vi "相对偏差百分比出数.vi"(0 "基准值":dbl, 2 "原始值":dbl, 3 "相对偏差百分比":dbl) -> (6 "取值输出":dbl, 7 "随机数？":bool)   [LabVIEW 2016, in "random number.lvlib"]
uses:
  random number.lvlib
panel:
  out "下限":dbl
  out "上限":dbl
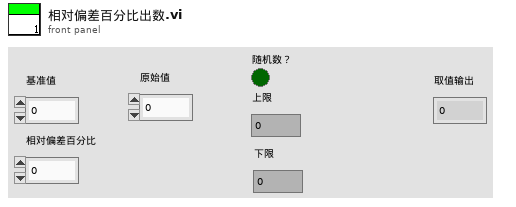
[diagram p1: front panel]
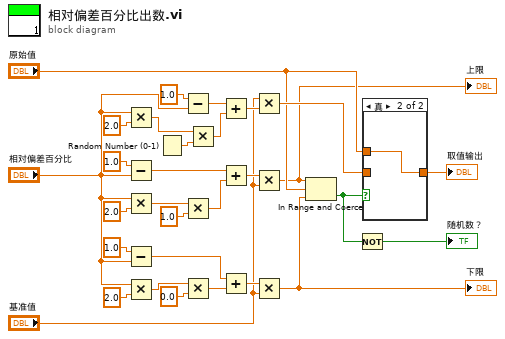
[diagram p0: block diagram]
diagram:
  n1 = Multiply(x="相对偏差百分比", y=2.0) -> (x*y=w23:dbl)
  n2 = Subtract(x=1.0, y="相对偏差百分比") -> (x-y=w12:dbl)
  n3 = Multiply(x="相对偏差百分比", y=2.0) -> (x*y=w11:dbl)
  n4 = Subtract(x=1.0, y="相对偏差百分比") -> (x-y=w21:dbl)
  n5 = Multiply(x="相对偏差百分比", y=2.0) -> (x*y=w22:dbl)
  n6 = Random Number (0-1)() -> (number: 0 to 1=w29:dbl)
  n7 = Subtract(x=1.0, y="相对偏差百分比") -> (x-y=w26:dbl)
  n8 = Multiply(x=w11, y=1.0) -> (x*y=w13:dbl)
  n9 = Multiply(x=w22, y=0.0) -> (x*y=w20:dbl)
  n10 = Multiply(x=w23, y=w29) -> (x*y=w27:dbl)
  n11 = Add(x=w26, y=w27) -> (x+y=w25:dbl)
  n12 = Add(x=w12, y=w13) -> (x+y=w9:dbl)
  n13 = Add(x=w21, y=w20) -> (x+y=w8:dbl)
  n14 = Multiply(x="基准值", y=w25) -> (x*y=w24:dbl)
  n15 = Multiply(x=w9, y="基准值") -> (x*y=w3:dbl)
  "上限" <- w3
  n16 = Multiply(x=w8, y="基准值") -> (x*y=w2:dbl)
  "下限" <- w2
  n17 = In Range and Coerce(upper limit=w3, x="原始值", lower limit=w2) -> (In Range?=w5:bool)  [unwired: 1 out]
  n18 = Not(x=w5) -> (.not. x?=→"随机数？":bool)
  n19 = case shown="真" w5 {
    tunnel: w24 -> [w31 _]
    tunnel: "原始值" -> [_ w32]
    tunnel: [w31 w32] -> w6
    frame False {
    }
    frame True {
    }
  }
  "取值输出" <- w6
